vi "initFile.vi"(11 "Init File":path=path "C:/Users/Administrator/Desktop/micro.ini") -> ()   [LabVIEW 2016]
uses:
  variables/configDB.vi
  <vilib>/Utility/config.llb/Read Key (I32).vi
  <vilib>/Utility/config.llb/Read Key (Double).vi
  <vilib>/Utility/config.llb/Read Key (String).vi
  variables/imageSettings.vi
  <vilib>/Utility/config.llb/NI_LVConfig.lvlib
panel:
  out "stageOrigin":string
  out "stageDivision":string
  out "yRange":dbl
  out "focalLength":dbl
  out "distance":dbl
  out "floatingDigits":i32
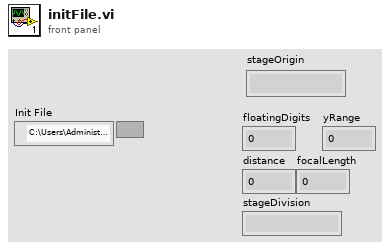
[diagram p1: front panel]
types:
  T1 = typedef "NI_LVConfig.lvlib/Config Data RefNum.ctl" = refnum<k1>
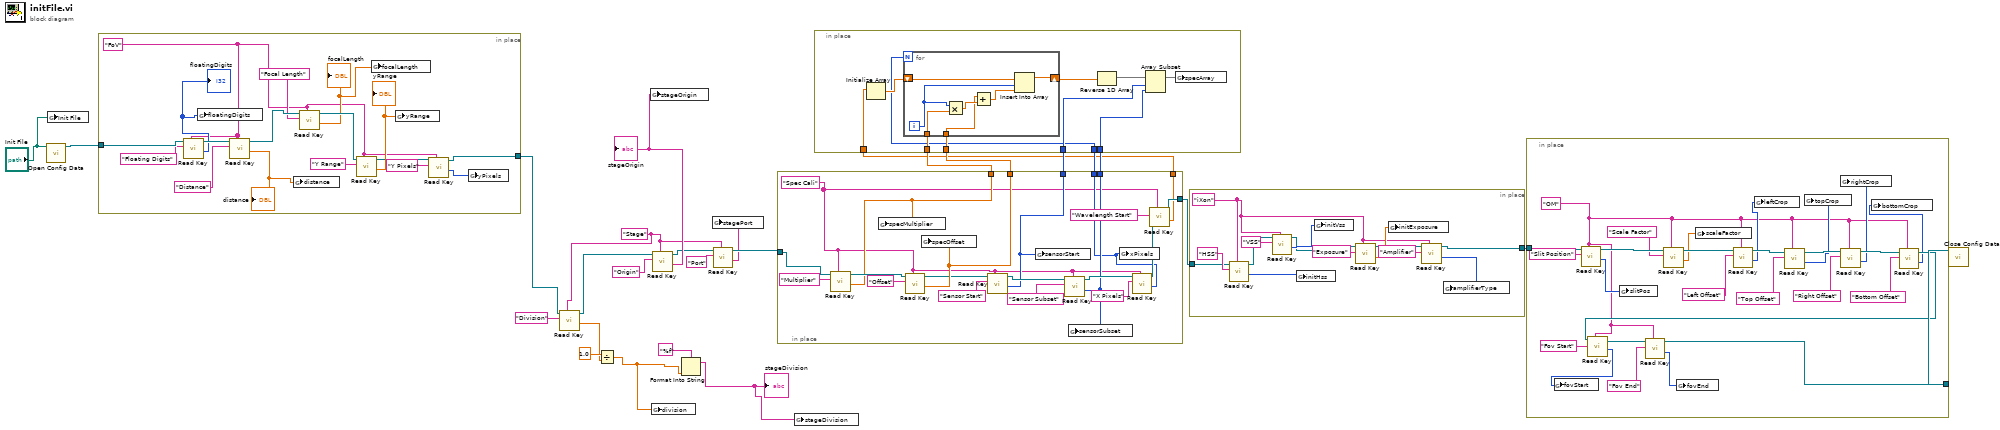
[diagram p0: block diagram]
diagram:
  w8 = "Stage" ("section")
  n1 = call <vilib>:"Open Config Data.vi"("configuration file path"="Init File") -> ("refnum"=w26:T1)  [unwired: 8 in, 2 out]
  n2 = global write "configDB.vi" "Init File"("Init File") -> ()
  n3 = in-place {
    in-place-border: w26 -> [w43]
    in-place-border: [w30] -> w25
    w28 = "FoV" ("section")
    n4 = call-poly <vilib>:"Read Key.vi"("section"=w28, "key"="Floating Digits", "refnum"=w43) -> ("value"=w32:i32, "refnum out"=w37:T1)  [unwired: 5 in, 2 out]
    "floatingDigits" <- w32
    n5 = global write "configDB.vi" "floatingDigits"(w32) -> ()
    n6 = call-poly <vilib>:"Read Key.vi"("section"=w28, "key"="Distance", "refnum"=w37) -> ("value"=w33:dbl, "refnum out"=w41:T1)  [unwired: 5 in, 2 out]
    "distance" <- w33
    n7 = global write "configDB.vi" "distance"(w33) -> ()
    n8 = call-poly <vilib>:"Read Key.vi"("section"=w28, "key"="Focal Length", "refnum"=w41) -> ("value"=w34:dbl, "refnum out"=w39:T1)  [unwired: 5 in, 2 out]
    "focalLength" <- w34
    n9 = call-poly <vilib>:"Read Key.vi"("section"=w28, "key"="Y Range", "refnum"=w39) -> ("value"=w35:dbl, "refnum out"=w31:T1)  [unwired: 5 in, 2 out]
    "yRange" <- w35
    n10 = global write "configDB.vi" "focalLength"(w34) -> ()
    n11 = global write "configDB.vi" "yRange"(w35) -> ()
    n12 = call-poly <vilib>:"Read Key.vi"("section"=w28, "key"="Y Pixels", "refnum"=w31) -> ("value"=w27:i32, "refnum out"=w30:T1)  [unwired: 5 in, 2 out]
    n13 = global write "configDB.vi" "yPixels"(w27) -> ()
  }
  n14 = call-poly <vilib>:"Read Key.vi"("section"=w8, "key"="Division", "refnum"=w25) -> ("value"=w22:dbl, "refnum out"=w17:T1)  [unwired: 5 in, 2 out]
  n15 = Divide(x=1.0, y=w22) -> (x/y=w19:dbl)
  n16 = global write "configDB.vi" "division"(w19) -> ()
  n17 = call-poly <vilib>:"Read Key.vi"("section"=w8, "key"="Origin", "refnum"=w17) -> ("value"=w16:string, "refnum out"=w11:T1)  [unwired: 5 in, 2 out]
  "stageOrigin" <- w16
  n18 = global write "configDB.vi" "stageOrigin"(w16) -> ()
  n19 = Format Into String(format string="%f", w19) -> (resulting string=w20:string)  [unwired: 2 in, 1 out]
  "stageDivision" <- w20
  n20 = call-poly <vilib>:"Read Key.vi"("section"=w8, "key"="Port", "refnum"=w11) -> ("value"=w7:string, "refnum out"=w10:T1)  [unwired: 5 in, 2 out]
  n21 = global write "configDB.vi" "stagePort"(w7) -> ()
  n22 = in-place {
    in-place-border: w10 -> [w63]
    in-place-border: [w59] -> w15
    in-place-border: [w58] -> w14
    in-place-border: [w47] -> w13
    in-place-border: [w52] -> w4
    in-place-border: [w51] -> w3
    in-place-border: [w48] -> w2
    in-place-border: [w44] -> w1
    w46 = "Spec Cali" ("section")
    n23 = call-poly <vilib>:"Read Key.vi"("section"=w46, "key"="Multiplier", "refnum"=w63) -> ("value"=w59:dbl, "refnum out"=w60:T1)  [unwired: 5 in, 2 out]
    n24 = global write "configDB.vi" "specMultiplier"(w59) -> ()
    n25 = call-poly <vilib>:"Read Key.vi"("section"=w46, "key"="Offset", "refnum"=w60) -> ("value"=w58:dbl, "refnum out"=w57:T1)  [unwired: 5 in, 2 out]
    n26 = global write "configDB.vi" "specOffset"(w58) -> ()
    n27 = call-poly <vilib>:"Read Key.vi"("section"=w46, "key"="Sensor Start", "refnum"=w57) -> ("value"=w52:i32, "refnum out"=w55:T1)  [unwired: 5 in, 2 out]
    n28 = global write "configDB.vi" "sensorStart"(w52) -> ()
    n29 = call-poly <vilib>:"Read Key.vi"("section"=w46, "key"="Sensor Subset", "refnum"=w55) -> ("value"=w51:i32, "refnum out"=w53:T1)  [unwired: 5 in, 2 out]
    n30 = global write "configDB.vi" "sensorSubset"(w51) -> ()
    n31 = call-poly <vilib>:"Read Key.vi"("section"=w46, "key"="X Pixels", "refnum"=w53) -> ("value"=w48:i32, "refnum out"=w50:T1)  [unwired: 5 in, 2 out]
    n32 = global write "configDB.vi" "xPixels"(w48) -> ()
    n33 = call-poly <vilib>:"Read Key.vi"("section"=w46, "key"="Wavelength Start", "refnum"=w50) -> ("value"=w44:dbl, "refnum out"=w47:T1)  [unwired: 5 in, 2 out]
  }
  n34 = global write "configDB.vi" "stageDivision"(w20) -> ()
  n35 = in-place {
    in-place-border: w15 -> [w71]
    in-place-border: w14 -> [w70]
    in-place-border: w4 -> [w67]
    in-place-border: w3 -> [w66]
    in-place-border: w2 -> [w65]
    in-place-border: w1 -> [w64]
    n36 = Initialize Array(w64) -> (w72:dbl[])  [unwired: 1 in]
    n37 = for {
      N: w65 -> [_]
      shift-right: [w79] -> w73
      shift-left: w72 -> [w80]
      tunnel: w71 -> [w74]
      tunnel: w70 -> [w75]
      i -> [w78]
      n38 = Multiply(x=w78, y=w74) -> (x*y=w77:dbl)
      n39 = Add(x=w75, y=w77) -> (x+y=w76:dbl)
      n40 = Insert Into Array(array=w80, index=w78, new element=w76) -> (w79:dbl[])
    }
    n41 = Reverse 1D Array(array=w73) -> (reversed array=w69:dbl[])
    n42 = Array Subset(array=w69, index=w67, length=w66) -> (w68:dbl[])
    n43 = global write "imageSettings.vi" "specArray"(w68) -> ()
  }
  n44 = in-place {
    in-place-border: [w84] -> w6
    in-place-border: w13 -> [w86]
    w83 = "iXon" ("section")
    n45 = call-poly <vilib>:"Read Key.vi"("section"=w83, "key"="HSS", "refnum"=w86) -> ("value"=w90:i32, "refnum out"=w93:T1)  [unwired: 5 in, 2 out]
    n46 = call-poly <vilib>:"Read Key.vi"("section"=w83, "key"="VSS", "refnum"=w93) -> ("value"=w91:i32, "refnum out"=w89:T1)  [unwired: 5 in, 2 out]
    n47 = global write "configDB.vi" "initHss"(w90) -> ()
    n48 = global write "configDB.vi" "initVss"(w91) -> ()
    n49 = call-poly <vilib>:"Read Key.vi"("section"=w83, "key"="Exposure", "refnum"=w89) -> ("value"=w87:dbl, "refnum out"=w85:T1)  [unwired: 5 in, 2 out]
    n50 = global write "configDB.vi" "initExposure"(w87) -> ()
    n51 = call-poly <vilib>:"Read Key.vi"("section"=w83, "key"="Amplifier", "refnum"=w85) -> ("value"=w81:i32, "refnum out"=w84:T1)  [unwired: 5 in, 2 out]
    n52 = global write "configDB.vi" "amplifierType"(w81) -> ()
  }
  n53 = in-place {
    in-place-border: w6 -> [w120]
    in-place-border: [w99] -> w5
    w98 = "OM" ("section")
    n54 = call-poly <vilib>:"Read Key.vi"("section"=w98, "key"="Slit Position", "refnum"=w120) -> ("value"=w114:i32, "refnum out"=w119:T1)  [unwired: 5 in, 2 out]
    n55 = global write "configDB.vi" "slitPos"(w114) -> ()
    n56 = call-poly <vilib>:"Read Key.vi"("section"=w98, "key"="Scale Factor", "refnum"=w119) -> ("value"=w115:dbl, "refnum out"=w117:T1)  [unwired: 5 in, 2 out]
    n57 = global write "configDB.vi" "scaleFactor"(w115) -> ()
    n58 = call-poly <vilib>:"Read Key.vi"("section"=w98, "key"="Left Offset", "refnum"=w117) -> ("value"=w105:i32, "refnum out"=w113:T1)  [unwired: 5 in, 2 out]
    n59 = global write "configDB.vi" "leftCrop"(w105) -> ()
    n60 = call-poly <vilib>:"Read Key.vi"("section"=w98, "key"="Top Offset", "refnum"=w113) -> ("value"=w104:i32, "refnum out"=w112:T1)  [unwired: 5 in, 2 out]
    n61 = global write "configDB.vi" "topCrop"(w104) -> ()
    n62 = call-poly <vilib>:"Read Key.vi"("section"=w98, "key"="Right Offset", "refnum"=w112) -> ("value"=w103:i32, "refnum out"=w111:T1)  [unwired: 5 in, 2 out]
    n63 = global write "configDB.vi" "rightCrop"(w103) -> ()
    n64 = call-poly <vilib>:"Read Key.vi"("section"=w98, "key"="Bottom Offset", "refnum"=w111) -> ("value"=w102:i32, "refnum out"=w110:T1)  [unwired: 5 in, 2 out]
    n65 = call-poly <vilib>:"Read Key.vi"("section"=w98, "key"="Fov Start", "refnum"=w110) -> ("value"=w96:i32, "refnum out"=w101:T1)  [unwired: 5 in, 2 out]
    n66 = global write "configDB.vi" "fovStart"(w96) -> ()
    n67 = call-poly <vilib>:"Read Key.vi"("section"=w98, "key"="Fov End", "refnum"=w101) -> ("value"=w95:i32, "refnum out"=w99:T1)  [unwired: 5 in, 2 out]
    n68 = global write "configDB.vi" "fovEnd"(w95) -> ()
    n69 = global write "configDB.vi" "bottomCrop"(w102) -> ()
  }
  n70 = call <vilib>:"Close Config Data.vi"("refnum"=w5) -> ()  [unwired: 9 in, 2 out]
